vi "Step Die Test.vi"() -> ()   [LabVIEW 2017]
uses:
  <vilib>/Utility/error.llb/whitespace.ctl
panel:
  in  "OK Button":bool
  out "substring":string
  out "Error Out":errorcluster
  in  "Error In":errorcluster
  out "Read Position":string
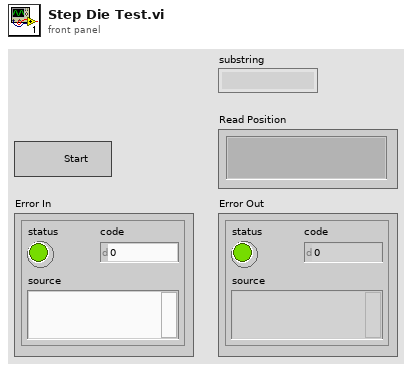
[diagram p1: front panel]
types:
  T1 = typedef "whitespace.ctl" = u16
  T2 = typedef "RegistrationNumber.ctl" = i32
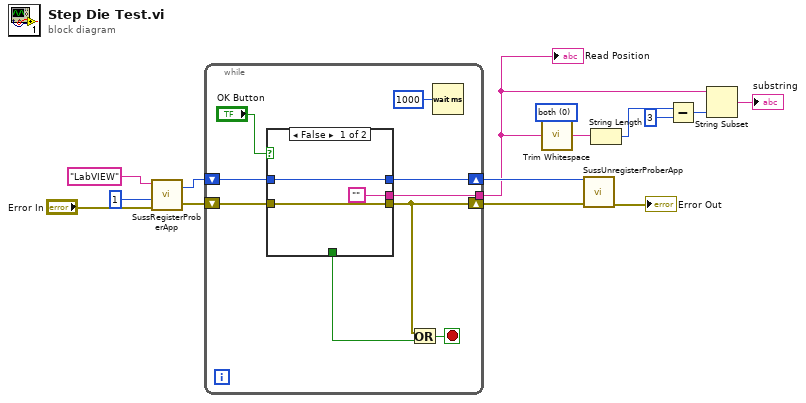
[diagram p0: block diagram]
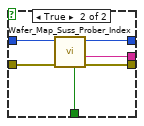
[diagram p2: hidden frame]
diagram:
  w8 = T1 0 items=["both", "start of string", "end of string"] ("location (both)")
  n1 = call <instrlib>:"SussRegisterProberApp.vi"("error in (no error)"="Error In", "Flag"=1, "Groupname"="LabVIEW") -> ("error out"=w13:errorcluster, "RegistrationNumber"=w1:T2)  [unwired: 1 in]
  n2 = while {
    tunnel: [w21] -> w2
    shift-right: [w19] -> w11
    shift-left: w13 -> [w24]
    shift-right: [w22] -> w12
    shift-left: w1 -> [w23]
    stop <- w20 stop-if-true
    n3 = case shown="False" "OK Button" {
      tunnel: w24 -> [w26 w33]
      tunnel: w23 -> [w27 w32]
      tunnel: [w27 w31] -> w22
      tunnel: [w26 w30] -> w19
      tunnel: ["" w29] -> w21
      tunnel: [_ w28] -> w18
      frame False {
      }
      frame True {
        n4 = call <instrlib>:"Wafer_Map_Suss_Prober_Index.vi"("error in (no error)"=w33, "RegistrationNumber"=w32) -> ("error out"=w30:errorcluster, "ResponseString 2"=w29:string, "RegistrationNumber out"=w31:T2, "End Of Wafer"=w28:bool)  [unwired: 6 in]
      }
    }
    n5 = Or(x=w19, y=w18) -> (x .or. y?=w20:bool)
    n6 = Wait (ms)(milliseconds to wait=u32 1000) -> ()  [unwired: 1 out]
  }
  "Read Position" <- w2
  n7 = call <vilib>:"Trim Whitespace.vi"("string"=w2, "location (both)"=w8) -> ("trimmed string"=w7:string)
  n8 = call <instrlib>:"SussUnregisterProberApp.vi"("error in"=w11, "RegistrationNumber"=w12) -> ("error out"=→"Error Out":errorcluster)  [unwired: 9 in]
  n9 = String Length(string=w7) -> (length=w5:i32)
  n10 = Subtract(x=w5, y=3) -> (x-y=w6:i32)
  n11 = String Subset(string=w2, length (rest)=w6) -> (substring=→"substring":string)  [unwired: 1 in]
